vi "events.get.vi"(11 "manager_daemon in":refnum<class "manager_daemon.lvclass">) -> (1 "display volume event":refnum<user-event>, 2 "refresh volume event":refnum<user-event>, 3 "manager_daemon out":refnum<class "manager_daemon.lvclass">)   [LabVIEW 2024, in "manager_daemon.lvclass"]
uses:
  manager_daemon.lvclass
  manager_daemon.lvclass/manager_daemon.ctl
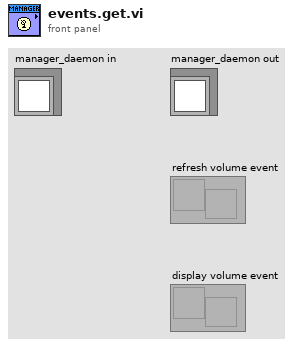
[diagram p1: front panel]
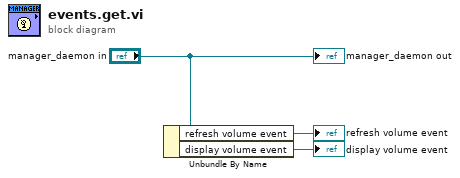
[diagram p0: block diagram]
diagram:
  n1 = Unbundle By Name("manager_daemon in") -> ("refresh volume event"=→"refresh volume event":refnum<user-event>, "display volume event"=→"display volume event":refnum<user-event>)
  "manager_daemon out" <- "manager_daemon in"
